vi "test filter by class.vi"() -> (3 "filter ok":bool)   [LabVIEW 2013, in "TBM Tests.lvlib"]
uses:
  TBM Tests.lvlib
  <vilib>/NI/Tag Bus/tag/tag descriptor.lvclass/tag descriptor.ctl
  channel/TBM channel.lvclass/TBM channel.ctl
  <vilib>/NI/Tag Bus/tag/read tag name.vi
  <vilib>/NI/Tag Bus/tag/read data type.vi
  channel/Read channel classification.vi
  channel/TBM channel.lvclass
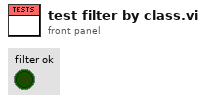
[diagram p1: front panel]
types:
  T1 = typedef "TBM channel.lvclass/channel classification.ctl" = enum16{"input data", "output data", "processing parameter", "processing result"}
  T2 = typedef "tag bus.lvlib/tag descriptor.lvclass/Data Type.ctl" = enum16{"Double", "Single", "I64", "I32", "I16", "I8", "U64", "U32", "U16", "U8", "Boolean", "String", "Array of Double", "Array of Single", "Array of I64", "Array of I32", "Array of I16", "Array of I8", "Array of U64", "Array of U32", "Array of U16", "Array of U8", "Array of Boolean", "Array of String"}
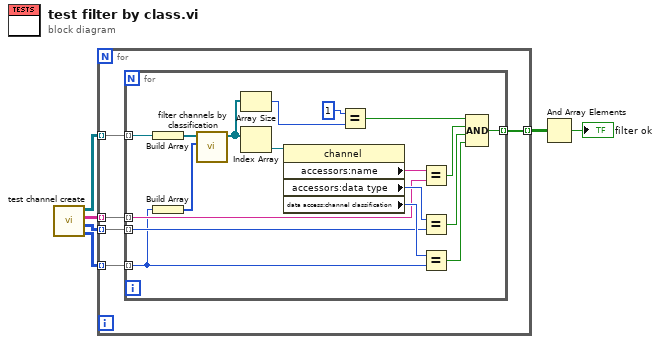
[diagram p0: block diagram]
diagram:
  n1 = call "test channel create.vi"() -> ("dirs"=w3:T1[][], "types"=w2:T2[][], "names"=w1:string[][], "chans"=w6:refnum<class "TBM channel.lvclass">[][])  [unwired: 5 in, 3 out]
  n2 = for {
    tunnel: w6 -> [w11] mode=indexing
    tunnel: w1 -> [w10] mode=indexing
    tunnel: [w9] -> w5 mode=indexing
    tunnel: w3 -> [w8] mode=indexing
    tunnel: w2 -> [w7] mode=indexing
    n3 = for {
      tunnel: w11 -> [w17] mode=indexing
      tunnel: w10 -> [w22] mode=indexing
      tunnel: [w26] -> w9 mode=indexing
      tunnel: w8 -> [w15] mode=indexing
      tunnel: w7 -> [w16] mode=indexing
      n4 = Build Array(w17) -> (w13:refnum<class "TBM channel.lvclass">[])
      n5 = Build Array(w15) -> (w14:T1[])
      n6 = call "filter channels by classification.vi"("allowed classifications"=w14, "channels in"=w13) -> ("channels out"=w12:refnum<class "TBM channel.lvclass">[])  [unwired: 9 in]
      n7 = Array Size(array=w12) -> (size(s)=w20:i32)
      n8 = Index Array(array=w12) -> (element=w21:refnum<class "TBM channel.lvclass">)  [unwired: 1 in]
      n9 = property class="channel"(reference=w21) -> ("accessors:name"=w25:string, "accessors:data type"=w24:T2, "data access:channel classification"=w23:T1)  [unwired: 1 in, 2 out]
      n10 = Equal?(x=1, y=w20) -> (x = y?=w18:bool)
      n11 = Equal?(x=w25, y=w22) -> (x = y?=w29:bool)
      n12 = Equal?(x=w24, y=w16) -> (x = y?=w28:bool)
      n13 = Equal?(x=w23, y=w15) -> (x = y?=w27:bool)
      n14 = Compound Arithmetic op=AND(w18, w29, w28, w27) -> (w26:bool)
    }
  }
  n15 = And Array Elements(Boolean array=w5) -> (logical AND=→"filter ok":bool)
